vi "Create Measurement.vi"(8 "error in (no error)":errorcluster, 10 "Measurement Name":string, 11 "XML Handler in":refnum<class "XML Handler.lvclass">) -> (0 "error out":errorcluster, 3 "XML Handler out":refnum<class "XML Handler.lvclass">)   [LabVIEW 2020, in "XML Handler.lvclass"]
uses:
  XML Handler.lvclass
  XML Handler.lvclass/XML Handler.ctl
  <vilib>/xml/Close Reference(Node).vi
  <resource>/objmgr/DOMUserDefRef.rc
  <vilib>/xml/NI_XML.lvlib
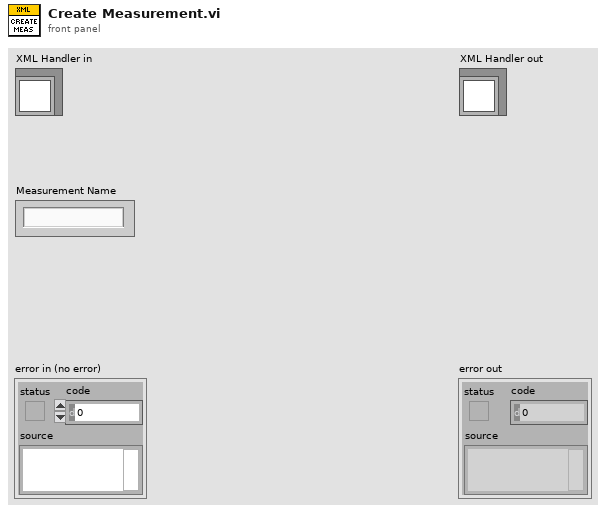
[diagram p1: front panel]
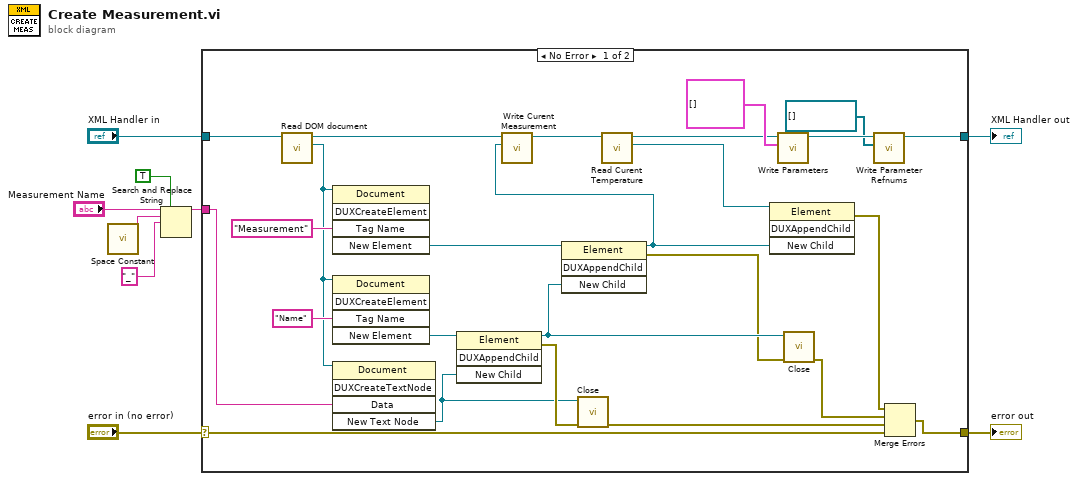
[diagram p0: block diagram]
diagram:
  n1 = call <vilib>:"Space Constant.vi"() -> ("String"=w2:string)
  n2 = Search and Replace String(replace all?=TRUE ("replace all? (F)"), input string="Measurement Name", search string=w2, replace string="_") -> (result string=w4:string)  [unwired: 4 in, 3 out]
  n3 = case shown="No Error" "error in (no error)" {
    selector: "error in (no error)" -> [w11 w36]
    tunnel: [w10 w36] -> w8
    tunnel: [w31 w35] -> w6
    tunnel: "XML Handler in" -> [w34 w35]
    tunnel: w4 -> [w26 _]
    frame No Error {
      n4 = call "Read DOM document.vi"("XML Handler in"=w34) -> ("DOM document"=w27:refnum<k20>, "XML Handler out"=w33:refnum<class "XML Handler.lvclass">)  [unwired: 9 in]
      n5 = invoke class="Document" method="DUXCreateElement"(reference=w27, "Tag Name"="Measurement") -> ("New Element"=w24:refnum<k20>)  [unwired: 3 in, 4 out]
      n6 = invoke class="Document" method="DUXCreateElement"(reference=w27, "Tag Name"="Name") -> ("New Element"=w25:refnum<k20>)  [unwired: 3 in, 4 out]
      n7 = invoke class="Document" method="DUXCreateTextNode"(reference=w27, "Data"=w26) -> ("New Text Node"=w22:refnum<k20>)  [unwired: 3 in, 4 out]
      n8 = invoke class="Element" method="DUXAppendChild"(reference=w25, "New Child"=w22) -> (reference out=w21:refnum<k20>, error out=w23:errorcluster)  [unwired: 2 in, 2 out]
      n9 = invoke class="Element" method="DUXAppendChild"(reference=w24, "New Child"=w21) -> (reference out=w15:refnum<k20>, error out=w20:errorcluster)  [unwired: 2 in, 2 out]
      n10 = call "Write Curent Measurement.vi"("Curent Measurement"=w15, "XML Handler in"=w33) -> ("XML Handler out"=w18:refnum<class "XML Handler.lvclass">)  [unwired: 9 in]
      n11 = call-poly <vilib>:"Close.vi"("error in (no error)"=w23, "node"=w22) -> ("error out"=w13:errorcluster)  [unwired: 7 in]
      n12 = call "Read Curent Temperature.vi"("XML Handler in"=w18) -> ("Curent Temperature"=w16:refnum<k20>, "XML Handler out"=w17:refnum<class "XML Handler.lvclass">)  [unwired: 9 in]
      n13 = invoke class="Element" method="DUXAppendChild"(reference=w16, "New Child"=w15) -> (error out=w14:errorcluster)  [unwired: 2 in, 3 out]
      n14 = call "Write Parameters.vi"("Parameters"=cluster{"Name":string, "Value":string}[] [], "XML Handler in"=w17) -> ("XML Handler out"=w32:refnum<class "XML Handler.lvclass">)  [unwired: 9 in]
      n15 = call-poly <vilib>:"Close.vi"("error in (no error)"=w20, "node"=w21) -> ("error out"=w12:errorcluster)  [unwired: 7 in]
      n16 = call "Write Parameter Refnums.vi"("Parameter Refnums"=refnum<k20>[] [], "XML Handler in"=w32) -> ("XML Handler out"=w31:refnum<class "XML Handler.lvclass">)  [unwired: 9 in]
      n17 = Merge Errors(w14, w12, w13, w11) -> (w10:errorcluster)
    }
    frame Error {
    }
  }
  "error out" <- w8
  "XML Handler out" <- w6
